vi "Constant - Default Serial Baud Rate.vi"() -> (3 "Baud Rate":i32=3000)   [LabVIEW 2021]
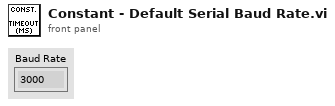
[diagram p1: front panel]
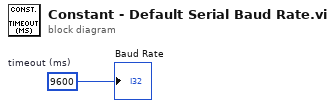
[diagram p0: block diagram]
diagram:
  w1 = 9600  # timeout (ms)
  "Baud Rate" <- w1
